vi "HFRR ADV v017 new software.vi"() -> ()   [LabVIEW 2025] (continued)
                        n2547 = Number To Fractional String(number=w3562, precision (6)=i16 2) -> (F-format string=w3561:string)  [unwired: 2 in]
                        n2548 = Concatenate Strings("Set Frequency [Hz] :" ("Content"), w3561) -> (w3564:string)
                        n2549 = local read "EVENT LOG"() -> (w3566:string)
                        n2550 = call "Event Log.vi"("Content"=w3564, "EVENT LOG"=w3566) -> ("EVENT LOG"=w3565:string)  [unwired: 8 in, 1 out]
                        n2551 = local write "EVENT LOG"(w3565) -> ()
                      }
                      frame #22 {
                        n2552 = Wait (ms)(milliseconds to wait=u32 50) -> ()  [unwired: 1 out]
                      }
                      frame #23 {
                        n2553 = local read "NORMAL LOAD"() -> (w3569:dbl)
                        n2554 = Number To Fractional String(number=w3569, precision (6)=i16 2) -> (F-format string=w3570:string)  [unwired: 2 in]
                        n2555 = Concatenate Strings("Applied Load [grams] :" ("Content"), w3570) -> (w3572:string)
                        n2556 = local read "EVENT LOG"() -> (w3574:string)
                        n2557 = call "Event Log.vi"("Content"=w3572, "EVENT LOG"=w3574) -> ("EVENT LOG"=w3573:string)  [unwired: 8 in, 1 out]
                        n2558 = local write "EVENT LOG"(w3573) -> ()
                      }
                      frame #24 {
                        n2559 = Wait (ms)(milliseconds to wait=u32 50) -> ()  [unwired: 1 out]
                      }
                      frame #25 {
                        n2560 = local read "Set Strk"() -> (w3577:dbl)
                        n2561 = Number To Fractional String(number=w3577, precision (6)=i16 2) -> (F-format string=w3578:string)  [unwired: 2 in]
                        n2562 = Concatenate Strings("Set Stroke [mm] :" ("Content"), w3578) -> (w3580:string)
                        n2563 = local read "EVENT LOG"() -> (w3582:string)
                        n2564 = call "Event Log.vi"("Content"=w3580, "EVENT LOG"=w3582) -> ("EVENT LOG"=w3581:string)  [unwired: 8 in, 1 out]
                        n2565 = local write "EVENT LOG"(w3581) -> ()
                      }
                      frame #26 {
                        n2566 = Wait (ms)(milliseconds to wait=u32 50) -> ()  [unwired: 1 out]
                      }
                      frame #27 {
                        n2567 = local read "Set Temp"() -> (w3585:dbl)
                        n2568 = Number To Fractional String(number=w3585, precision (6)=i16 2) -> (F-format string=w3586:string)  [unwired: 2 in]
                        n2569 = Concatenate Strings("Set Temperature [deg C] :" ("Content"), w3586) -> (w3588:string)
                        n2570 = local read "EVENT LOG"() -> (w3590:string)
                        n2571 = call "Event Log.vi"("Content"=w3588, "EVENT LOG"=w3590) -> ("EVENT LOG"=w3589:string)  [unwired: 8 in, 1 out]
                        n2572 = local write "EVENT LOG"(w3589) -> ()
                      }
                      frame #28 {
                        n2573 = Wait (ms)(milliseconds to wait=u32 50) -> ()  [unwired: 1 out]
                      }
                      frame #29 {
                        n2574 = local read "Set Rh"() -> (w3593:dbl)
                        n2575 = Number To Fractional String(number=w3593, precision (6)=i16 2) -> (F-format string=w3594:string)  [unwired: 2 in]
                        n2576 = Concatenate Strings("Set Humidity [%RH] :" ("Content"), w3594) -> (w3596:string)
                        n2577 = local read "EVENT LOG"() -> (w3598:string)
                        n2578 = call "Event Log.vi"("Content"=w3596, "EVENT LOG"=w3598) -> ("EVENT LOG"=w3597:string)  [unwired: 8 in, 1 out]
                        n2579 = local write "EVENT LOG"(w3597) -> ()
                      }
                      frame #30 {
                        n2580 = Wait (ms)(milliseconds to wait=u32 50) -> ()  [unwired: 1 out]
                      }
                      frame #31 {
                        n2581 = local read "test time"() -> (w3601:dbl)
                        n2582 = Number To Fractional String(number=w3601, precision (6)=i16 1) -> (F-format string=w3602:string)  [unwired: 2 in]
                        n2583 = Concatenate Strings("Test Duration [mins] :" ("Content"), w3602) -> (w3604:string)
                        n2584 = local read "EVENT LOG"() -> (w3606:string)
                        n2585 = call "Event Log.vi"("Content"=w3604, "EVENT LOG"=w3606) -> ("EVENT LOG"=w3605:string)  [unwired: 8 in, 1 out]
                        n2586 = local write "EVENT LOG"(w3605) -> ()
                      }
                      frame #32 {
                        w3607 = dbl[] [] ("History Data")
                        w3608 = cluster{"y":dbl, dbl, "y":dbl}[] [] ("History Data")
                        w3609 = FALSE ("Visible")
                        n2587 = property on="Stroke ( mm )" class="WFChart (strict)"("History Data"=w3608) -> ()  [unwired: 2 in, 2 out]
                        n2588 = property on="Humidity ( %RH )" class="WFChart (strict)"("History Data"=w3607) -> ()  [unwired: 2 in, 2 out]
                        n2589 = property on="Temperature ( Deg C )" class="WFChart (strict)"("History Data"=w3607) -> ()  [unwired: 2 in, 2 out]
                        n2590 = property on="Electrical Contact Resistance ( % )" class="WFChart (strict)"("History Data"=w3607) -> ()  [unwired: 2 in, 2 out]
                        n2591 = property on="Coefficient of Friction" class="WFChart (strict)"("History Data"=w3607) -> ()  [unwired: 2 in, 2 out]
                        n2592 = property on="Frictional Force ( N )" class="WFChart (strict)"("History Data"=w3607) -> ()  [unwired: 2 in, 2 out]
                        n2593 = property on="Coefficient of Friction" class="WFChart (strict)"("History Data"=w3607) -> ()  [unwired: 2 in, 2 out]
                        n2594 = property on="Frictional Force ( N )" class="WFChart (strict)"("History Data"=w3607) -> ()  [unwired: 2 in, 2 out]
                        n2595 = property on="Electrical Contact Resistance ( % )" class="WFChart (strict)"("History Data"=w3607) -> ()  [unwired: 2 in, 2 out]
                        n2596 = property on="Humidity ( %RH )" class="WFChart (strict)"("History Data"=w3607) -> ()  [unwired: 2 in, 2 out]
                        n2597 = property on="Stroke ( mm )" class="WFChart (strict)"("History Data"=w3608) -> ()  [unwired: 2 in, 2 out]
                        n2598 = property on="Temperature ( Deg C )" class="WFChart (strict)"("History Data"=w3607) -> ()  [unwired: 2 in, 2 out]
                        n2599 = property on="Service Password Log" class="Str"("Visible"=w3609) -> ()  [unwired: 2 in, 2 out]
                        n2600 = property on="Password 3" class="Clust (strict)"("Visible"=w3609) -> ()  [unwired: 2 in, 2 out]
                      }
                    }
                    "TEST FILE NAM,E SAVED" <- TRUE ("TEST FILE NAM,E SAVED")
                  }
                }
              }
            }
          }
        }
        n2601 = case shown="True" w2906 {
          frame False {
            n2602 = local write "tfalg"(0.0 ("tfalg")) -> ()
          }
          frame True {
            n2603 = local read "tfalg"() -> (w3051:dbl)
            n2604 = Equal?(x=w3051, y=0.0) -> (x = y?=w3052:bool)
            n2605 = case shown="True" w3052 {
              frame False {
              }
              frame True {
                n2606 = local read "Total No. of Tests"() -> (w3055:dbl)
                n2607 = local write "tfalg"(1.0 ("tfalg")) -> ()
                n2608 = local write "acq 2"(FALSE ("acq 2")) -> ()
                n2609 = Wait (ms)(milliseconds to wait=u32 200) -> ()  [unwired: 1 out]
                n2610 = Increment(x=w3055) -> (x+1=w3054:dbl)
                n2611 = local write "Total No. of Tests"(w3054) -> ()
              }
            }
          }
        }
        n2612 = local write "Test \nStatus"(w2912) -> ()
        n2613 = local write "Save"(w2912) -> ()
        n2614 = local read "Main Tab"() -> (w2869:T2)
        n2615 = case shown="True" w2893 {
          tunnel: [FALSE ("RUN") TRUE ("RUN")] -> w2892
          tunnel: [_ 1] -> w2885
          frame False {
          }
          frame True {
          }
        }
        n2616 = In Range and Coerce(upper limit=w2900, x=w2873, lower limit=w2899) -> (In Range?=w2891:bool)  [unwired: 1 out]
        n2617 = In Range and Coerce(upper limit=w2897, x=w2872, lower limit=w2898) -> (In Range?=w2889:bool)  [unwired: 1 out]
        n2618 = case shown="True" w2905 {
          frame False {
            n2619 = local read "Rt 3"() -> (w3033:bool)
            n2620 = case shown="True" w3033 {
              frame False {
              }
              frame True {
                n2621 = local write "Rt 3"(FALSE ("Rt 3")) -> ()
                n2622 = local write "Json End Flg"(TRUE ("Upld AR 2")) -> ()
              }
            }
            "Rt" <- TRUE ("Rt")
            "Rt 2" <- FALSE ("Rt")
          }
          frame True {
            n2623 = local read "Rt"() -> (w3040:bool)
            n2624 = local write "Rt 2"(TRUE ("Rt 2")) -> ()
            n2625 = case shown="True" w3040 {
              frame False {
              }
              frame True {
                w3041 = TRUE ("Upld AR 2")
                n2626 = local write "Rt"(FALSE ("Rt")) -> ()
                n2627 = local write "Upld AR"(w3041) -> ()
                n2628 = local write "Json St Flg"(w3041) -> ()
              }
            }
            "Rt 3" <- TRUE ("Rt 3")
          }
        }
        n2629 = case shown="True" w2891 {
          tunnel: [FALSE ("RUN") TRUE ("RUN")] -> w2890
          tunnel: [_ 2] -> w2884
          frame False {
          }
          frame True {
          }
        }
        n2630 = case shown="True" w2889 {
          tunnel: [FALSE ("RUN") TRUE ("RUN")] -> w2888
          tunnel: [_ 3] -> w2883
          frame False {
          }
          frame True {
          }
        }
        n2631 = case shown="\"Acquire\"" w2869 {
          tunnel: w2871 -> [_ w3102]
          frame Default {
            w3101 = 0.0 ("output")
            n2632 = local write "PID-out"(w3101) -> ()
            n2633 = local write "Frequency ( Hz )"(w3101) -> ()
          }
          frame "Acquire" {
            n2634 = stacked-sequence {
              frame #0 {
                n2635 = local read "Auto Start Test"() -> (w3104:bool)
                n2636 = case shown="True" w3104 {
                  tunnel: "RUN" -> [w3125 w3128]
                  tunnel: [w3125 w3127] -> w3105
                  frame False {
                  }
                  frame True {
                    n2637 = local read "Auto Start Temp"() -> (w3126:bool)
                    n2638 = Or(x=w3128, y=w3126) -> (x .or. y?=w3127:bool)
                  }
                }
                n2639 = local read "clk"() -> (w3124:dbl)
                n2640 = local read "Save"() -> (w3120:bool)
                n2641 = Equal?(x=w3124, y=0.0) -> (x = y?=w3121:bool)
                n2642 = And(x=w3121, y=w3120) -> (x .and. y?=w3122:bool)
                n2643 = Not(x="Engage") -> (.not. x?=w3111:bool)
                n2644 = case shown="False" w3105 {
                  tunnel: [0.0 w3151] -> w3107
                  frame False {
                    (unwired) TRUE ("Visible")
                    n2645 = local read "Auto Start Test"() -> (w3132:bool)
                    n2646 = local write "Start Time"(TRUE ("Start Time")) -> ()
                    n2647 = property on="Stroke 2" class="DigNum (strict)"("Visible"=FALSE) -> ()  [unwired: 2 in, 2 out]
                    n2648 = case shown="False" w3132 {
                      frame False {
                        n2649 = property on="Heater Button" class="Bool (strict)"("DisabledEnum"=T19."Enabled" ("Disabled")) -> ()  [unwired: 2 in, 2 out]
                        n2650 = property on="Humidity" class="Bool (strict)"("DisabledEnum"=T19."Enabled" ("Disabled")) -> ()  [unwired: 2 in, 2 out]
                      }
                      frame True {
                      }
                    }
                    n2651 = case shown="False" "TestCompFlg" {
                      frame False {
                        n2652 = local read "StartFlg"() -> (w3140:bool)
                        n2653 = case shown="True" w3140 {
                          frame False {
                          }
                          frame True {
                            n2654 = stacked-sequence {
                              frame #0 {
                                n2655 = local read "EVENT LOG"() -> (w3144:string)
                                n2656 = call "Event Log.vi"("Content"="Test was interrupted", "EVENT LOG"=w3144) -> ("EVENT LOG"=w3145:string)  [unwired: 8 in, 1 out]
                                n2657 = local write "EVENT LOG"(w3145) -> ()
                                n2658 = property on="RUN" class="Bool (strict)"("Visible"=TRUE) -> ()  [unwired: 2 in, 2 out]
                                n2659 = property on="Auto Start Test" class="Bool (strict)"("Visible"=TRUE) -> ()  [unwired: 2 in, 2 out]
                              }
                              frame #1 {
                                w3147 = FALSE ("StartFlg")
                                n2660 = property on="Heater Button" class="Bool (strict)"("Val(Sgnl)"=FALSE ("Value (Signaling)")) -> ()  [unwired: 2 in, 2 out]
                                n2661 = local write "Heater Button"(w3147) -> ()
                                n2662 = local write "StartFlg"(w3147) -> ()
                                n2663 = local write "Humidity"(w3147) -> ()
                              }
                              frame #2 {
                                n2664 = local write "Command"("VC;0" ("Command")) -> ()
                              }
                              frame #3 {
                                n2665 = Wait (ms)(milliseconds to wait=u32 1500) -> ()  [unwired: 1 out]
                              }
                              frame #4 {
                                n2666 = local write "Command"("HE;0" ("Command")) -> ()
                              }
                            }
                          }
                        }
                      }
                      frame True {
                      }
                    }
                    n2667 = local write "String 14"("Test will autostart once parameters reach the set value." ("String 14")) -> ()
                  }
                  frame True {
                    (unwired) FALSE ("Visible")
                    n2668 = property on="Stroke 2" class="DigNum (strict)"("Visible"=TRUE) -> ()  [unwired: 2 in, 2 out]
                    n2669 = property on="STOP 2" class="Bool (strict)"("Disabled"=u8 2) -> ()  [unwired: 2 in, 2 out]
                    n2670 = local write "String 14"(" Running....." ("String 14")) -> ()
                    n2671 = property on="Heater Button" class="Bool (strict)"("DisabledEnum"=T19."Disabled and Grayed Out" ("Disabled")) -> ()  [unwired: 2 in, 2 out]
                    n2672 = property on="Humidity" class="Bool (strict)"("DisabledEnum"=T19."Disabled and Grayed Out" ("Disabled")) -> ()  [unwired: 2 in, 2 out]
                    n2673 = case shown="True" "Start Time" {
                      selector: "Start Time" -> [_ w3170]
                      frame False {
                      }
                      frame True {
                        n2674 = Not(x=w3170) -> (.not. x?=w3169:bool)
                        n2675 = local write "Start Time"(w3169) -> ()
                        n2676 = local read "EVENT LOG"() -> (w3171:string)
                        n2677 = call "Event Log.vi"("Content"="Test in progress", "EVENT LOG"=w3171) -> ("EVENT LOG"=w3173:string)  [unwired: 8 in, 1 out]
                        n2678 = local write "EVENT LOG"(w3173) -> ()
                      }
                    }
                    n2679 = disable-structure shown="Enabled" {
                      disable-tunnel: [w3162 w3168] -> w3151
                      frame Disabled {
                        n2680 = local read "Set Hz"() -> (w3165:dbl)
                        n2681 = call <vilib>:"Uniform White Noise Waveform.vi"() -> ("signal out"=w3164:waveform(dbl))  [unwired: 10 in, 1 out]
                        n2682 = Random Number (0-1)() -> (number: 0 to 1=w3161:dbl)
                        n2683 = Add(x=w3165, y=w3164) -> (x+y=w3163:waveform(dbl))
                        n2684 = Multiply(x=ext 0.01 ("y"), y=w3161) -> (x*y=w3159:ext)
                        n2685 = Multiply(x=w3163, y=w3159) -> (x*y=w3162:waveform(ext))
                      }
                      frame Enabled {
                        n2686 = call-poly <vilib>:"Random Number (Range).vi"("lower bound (0)"=49.89, "upper bound (100)"=50.8) -> ("number"=w3168:dbl)  [unwired: 9 in]
                      }
                    }
                    "StartFlg" <- TRUE ("StartFlg")
                  }
                }
                n2687 = case shown="True" w3122 {
                  frame False {
                  }
                  frame True {
                    n2688 = local write "clk"(10.0 ("clk")) -> ()
                    n2689 = Get Date/Time In Seconds() -> (seconds since 1Jan1904=w3176:timestamp)
                    n2690 = To Double Precision Float(number=w3176) -> (double precision float=w3174:dbl)
                    n2691 = local write "acq timer"(w3174) -> ()
                    n2692 = local write "act save time"(w3174) -> ()
                  }
                }
                n2693 = call "Elapsed Time"("Time Target (s)"="Countdown", "Reset"=w3111) -> ("Elapsed Time (s)"=w3116:dbl, "Time has Elapsed"=w3114:bool)  [unwired: 10 in, 6 out]
                "Countdown 2" <- w3116
                n2694 = Subtract(x=w3116, y=2.0) -> (x-y=w3119:dbl)
                n2695 = Less?(x=w3119, y="Countdown") -> (x < y?=w3117:bool)
                n2696 = And(x=w3117, y=w3114) -> (x .and. y?=w3113:bool)
                n2697 = case shown="True" w3113 {
                  frame False {
                  }
                  frame True {
                    (unwired) dbl[] [] ("History Data")
                    n2698 = local write "Engage"(FALSE ("Engage")) -> ()
                    n2699 = local write "RUN"(TRUE ("RUN")) -> ()
                    n2700 = local read "Humidity ( %RH )"() -> (→"Rh Before":dbl)
                  }
                }
                n2701 = local read "Test \nStatus"() -> (w3109:bool)
                n2702 = Select(t=w3107, s=w3109, f=0.0) -> (s? t:f=w3108:dbl)
                n2703 = local write "Frequency ( Hz )"(w3108) -> ()
              }
              frame #1 {
                w3199 = 1000000.0 ("x")
                # "HC;1/0\nST;VALUE"
                # "Elapsed time\ncof\nstroke\nAir temp\nTemp\nHumidity"
                # "acq timer\n\nact save time"
                # "convert to microseconds"
                n2704 = local read "COUNT"() -> (w3182:i32)
                n2705 = local read "Rate"() -> (w3195:dbl)
                n2706 = Divide(x=w3199, y=w3195) -> (x/y=w3200:dbl)
                n2707 = Greater Or Equal?(x=w3182, y=250) -> (x >= y?=w3181:bool)
                n2708 = Get Date/Time In Seconds() -> (seconds since 1Jan1904=w3202:timestamp)
                n2709 = case shown="True" w3181 {
                  frame False {
                    n2710 = local read "COUNT"() -> (w3203:i32)
                    n2711 = Increment(x=w3203) -> (x+1=w3204:i32)
                    n2712 = local write "COUNT"(w3204) -> ()
                  }
                  frame True {
                    n2713 = local write "COUNT"(0 ("COUNT")) -> ()
                  }
                }
                n2714 = local read "Samplingtime 2"() -> (w3180:dbl)
                n2715 = local read "act save time"() -> (w3197:dbl)
                n2716 = Divide(x=w3200, y=w3199) -> (x/y=w3198:dbl)
                n2717 = To Double Precision Float(number=w3202) -> (double precision float=w3191:dbl)
                n2718 = Add(x=w3197, y=w3180) -> (x+y=w3196:dbl)
                n2719 = local read "acq timer"() -> (w3201:dbl)
                n2720 = local read "COUNT"() -> (w3184:i32)
                n2721 = Greater Or Equal?(x=w3191, y=w3196) -> (x >= y?=w3179:bool)
                n2722 = Multiply(x=w3198, y=w3184) -> (x*y=w3190:dbl)
                n2723 = Subtract(x=w3191, y=w3201) -> (x-y=w3193:dbl)
                n2724 = local read "Save"() -> (w3194:bool)
                n2725 = Add(x=w3193, y=w3190) -> (x+y=w3177:dbl)
                "Elapsed time 3" <- w3177
                n2726 = And(x=w3179, y=w3194) -> (x .and. y?=w3192:bool)
                n2727 = Divide(x=w3177, y=60.0) -> (x/y=w3188:dbl)
                n2728 = local read "Test \nStatus"() -> (w3178:bool)
                n2729 = local read "clk"() -> (w3185:dbl)
                n2730 = Equal?(x=w3185, y=10.0) -> (x = y?=w3187:bool)
                n2731 = case shown="True" w3192 {
                  tunnel: w3191 -> [_ w3315]
                  tunnel: [FALSE ("Boolean 2") TRUE ("Boolean 2")] -> _
                  frame False {
                  }
                  frame True {
                    w3269 = ";" ("Substring")
                    # "Pid out/\nFreq response value"
                    n2732 = local write "act save time"(w3315) -> ()
                    n2733 = local read "FILE"() -> (w3263:string)
                    n2734 = call "file check.vi"("file name in"=w3263) -> ("error out"=w3266:errorcluster, "file name out"=w3261:string)  [unwired: 9 in]
                    n2735 = local read "LVDT STROKE"() -> (w3258:dbl)
                    n2736 = local read "Add up Stroke"() -> (w3256:dbl)
                    n2737 = call "FILE PATH CREATION.vi"("error in"=w3266, "FILE NAME :"=w3261) -> ("FILE OUT"=w3264:path)  [unwired: 8 in, 1 out]
                    n2738 = Concatenate Strings(w3261, ".dgf" ("Substring")) -> (w3265:string)
                    n2739 = Subtract(x=w3258, y=w3256) -> (x-y=w3257:dbl)
                    n2740 = Absolute Value(x=w3257) -> (abs(x)=w3255:dbl)
                    n2741 = local read "FF 2"() -> (→"Frictional Force ( N )" →"Frictional Force ( N )":dbl)
                    n2742 = Build Path(base path=w3264, name or relative path=w3265) -> (appended path=w3260:path)
                    n2743 = local read "COF 2"() -> (w3274:dbl)
                    "cof" <- w3274
                    "Coefficient of Friction" <- w3274
                    "COF 4" <- w3274
                    "Coefficient of Friction" <- w3274
                    n2744 = local read "TEMP"() -> (w3277:dbl)
                    "Temp" <- w3277
                    "Temperature ( Deg C )" <- w3277
                    n2745 = local read "Humidity ( %RH )"() -> (w3276:dbl)
                    "Humidity ( %RH )" <- w3276
                    "Humidity ( %RH )" <- w3276
                    n2746 = local read "Frequency ( Hz )"() -> (w3283:dbl)
                    n2747 = call <vilib>:"Mean PtByPt.vi"("x"=w3255, "sample length"="STROKE FILTER") -> ("mean"=w3254:dbl)  [unwired: 2 in, 1 out]
                    n2748 = local read "Elapsed time"() -> (w3308:dbl)
                    n2749 = local read "AIR TEMP"() -> (w3281:dbl)
                    n2750 = local read "PID-out"() -> (w3286:dbl)
                    n2751 = local write "Temperature ( Deg C )"(w3277) -> ()
                    n2752 = Number To Fractional String(number=w3254, width (-)=i16 9 ("precision (6)"), precision (6)=i16 6) -> (F-format string=w3301:string)  [unwired: 1 in]
                    n2753 = Number To Fractional String(number=w3281, width (-)=i16 9 ("precision (6)"), precision (6)=i16 3) -> (F-format string=w3300:string)  [unwired: 1 in]
                    n2754 = Number To Fractional String(number=w3277, width (-)=i16 9 ("precision (6)"), precision (6)=i16 3) -> (F-format string=w3297:string)  [unwired: 1 in]
                    n2755 = Number To Fractional String(number=w3276, width (-)=i16 9 ("precision (6)"), precision (6)=i16 3) -> (F-format string=w3294:string)  [unwired: 1 in]
                    n2756 = Number To Fractional String(number=0.0, width (-)=i16 9 ("precision (6)"), precision (6)=i16 3) -> (F-format string=w3291:string)  [unwired: 1 in]
                    n2757 = Number To Fractional String(number=w3286, width (-)=i16 9 ("precision (6)"), precision (6)=i16 3) -> (F-format string=w3287:string)  [unwired: 1 in]
                    n2758 = Number To Fractional String(number=w3283, width (-)=i16 9 ("precision (6)"), precision (6)=i16 3) -> (F-format string=w3282:string)  [unwired: 1 in]
                    n2759 = Number To Fractional String(number=w3274, width (-)=i16 9 ("precision (6)"), precision (6)=i16 6) -> (F-format string=w3309:string)  [unwired: 1 in]
                    n2760 = Number To Fractional String(number=w3308, width (-)=i16 14 ("precision (6)"), precision (6)=i16 3) -> (F-format string=w3310:string)  [unwired: 1 in]
                    n2761 = Bundle("y"=1.02, "mean"=w3254, "y"=0.98) -> (w3275:cluster{"y":dbl, "mean":dbl, "y":dbl})  [unwired: 1 in]
                    n2762 = Number To Fractional String(number="Ambient Humidity :", width (-)=i16 9 ("precision (6)"), precision (6)=i16 6) -> (F-format string=w3267:string)  [unwired: 1 in]
                    n2763 = local read "RUN"() -> (w3273:bool)
                    n2764 = case shown="True" w3273 {
                      tunnel: w3275 -> [_ w3320]
                      tunnel: w3254 -> [_ w3319]
                      tunnel: w3254 -> [_ w3317]
                      tunnel: w3254 -> [_ w3318]
                      frame False {
                      }
                      frame True {
                        "Stroke ( mm )" <- w3320
                        "Stroke ( mm )" <- w3320
                        "Stroke 4" <- w3319
                        "Stroke 3" <- w3317
                        "Stroke 2" <- w3318
                        "measured_stroke" <- w3317
                      }
                    }
                    n2765 = Concatenate Strings(w3310, w3269, w3309, w3269, w3301, w3269, w3300, w3269, w3297, w3269, w3294, w3269, w3291, w3269, w3287, w3269, w3282, w3269, w3267, "\r") -> (w3307:string)
                    n2766 = call <vilib>:"Write Characters To File.vi"("append to file? (new file:F)"=TRUE, "character string"=w3307, "file path (dialog if empty)"=w3260) -> ()  [unwired: 2 in, 1 out]
                    "refresh flag" <- TRUE ("refresh flag")
                  }
                }
                n2767 = case shown="True" w3178 {
                  tunnel: w3188 -> [_ w3214]
                  tunnel: w3193 -> [_ w3224]
                  tunnel: [0.0 w3220] -> _
                  tunnel: w3187 -> [_ w3219]
                  tunnel: [0.0 w3218] -> _
                  tunnel: w3177 -> [_ w3218]
                  tunnel: w3191 -> [w3207 _]
                  frame False {
                    n2768 = local write "acq timer"(w3207) -> ()
                    n2769 = local write "Test Duration Status"(0.0 ("Test Duration Status")) -> ()
                  }
                  frame True {
                    n2770 = local read "Set Hz"() -> (w3221:dbl)
                    n2771 = local write "Elapsed time"(w3214) -> ()
                    n2772 = local read "test time"() -> (w3213:dbl)
                    n2773 = Multiply(x=w3224, y=w3221) -> (x*y=w3223:dbl)
                    n2774 = case shown="False" w3219 {
                      tunnel: w3223 -> [w3225 _]
                      tunnel: [w3225 1.0] -> w3220
                      frame False {
                        n2775 = local write "Cycles elapsed"(w3225) -> ()
                      }
                      frame True {
                      }
                    }
                    n2776 = Greater?(x=w3214, y=w3213) -> (0:w3222:bool)
                    n2777 = Subtract(x=w3213, y=w3214) -> (x-y=w3212:dbl)
                    "time" <- w3212
                    n2778 = Multiply(x=w3212, y=60.0) -> (x*y=w3211:dbl)
                    n2779 = local write "Time Remaining"(w3211) -> ()
                    n2780 = local write "Remaining Time"(w3211) -> ()
                    n2781 = case shown="True" w3222 {
                      frame False {
                      }
                      frame True {
                        n2782 = stacked-sequence {
                          frame #0 {
                            w3230 = T19."Enabled" ("Disabled")
                            w3229 = FALSE ("TEST FILE NAM,E SAVED")
                            w3231 = "" ("FILE")
                            w3232 = TRUE ("Visible")
                            n2783 = local write "Humidity"(FALSE ("Humidity")) -> ()
                            n2784 = local write "RUN"(FALSE ("OK Button 2")) -> ()
                            n2785 = local write "Heater Button"(FALSE ("Heater Button")) -> ()
                            n2786 = local write "Auto Start Test"(FALSE ("Auto Start Test")) -> ()
                            n2787 = local write "TestCompFlg"(TRUE ("StpFlg")) -> ()
                            n2788 = local read "Humidity ( %RH )"() -> (→"Rh After":dbl)
                            n2789 = property on="STOP 2" class="Bool (strict)"("Disabled"=u8 0) -> ()  [unwired: 2 in, 2 out]
                            n2790 = local read "EVENT LOG"() -> (w3237:string)
                            n2791 = call "Event Log.vi"("Content"="Test Completed", "EVENT LOG"=w3237) -> ("EVENT LOG"=w3236:string)  [unwired: 8 in, 1 out]
                            n2792 = property on="RUN" class="Bool (strict)"("Visible"=w3232) -> ()  [unwired: 2 in, 2 out]
                            n2793 = property on="Auto Start Test" class="Bool (strict)"("Visible"=w3232) -> ()  [unwired: 2 in, 2 out]
                            n2794 = local write "Batch Ref Num :"(w3231) -> ()
                            n2795 = local write "FILE"(w3231) -> ()
                            n2796 = local write "EVENT LOG"(w3236) -> ()
                            n2797 = local write "TEST FILE NAM,E SAVED"(w3229) -> ()
                            n2798 = local write "Fuel Discription :"(w3231) -> ()
                            n2799 = local write "START TEMP"(w3229) -> ()
                            n2800 = local write "Remarks :"(w3231) -> ()
                            n2801 = local write "Main Dashboard Buttons"(T1."Imaging" ("Main Dashboard Buttons")) -> ()
                            n2802 = local write "Main Tab"(T2."Adv Scar" ("Main Tab")) -> ()
                            n2803 = property on="FRICVALZ 2" class="Bool (strict)"("DisabledEnum"=w3230) -> ()  [unwired: 2 in, 2 out]
                            n2804 = property on="FRICVALZ 3" class="Bool (strict)"("DisabledEnum"=w3230) -> ()  [unwired: 2 in, 2 out]
                            n2805 = property on="FRICVALZ 4" class="Bool (strict)"("DisabledEnum"=w3230) -> ()  [unwired: 2 in, 2 out]
                          }
                          frame #1 {
                            n2806 = Wait (ms)(milliseconds to wait=u32 1500) -> ()  [unwired: 1 out]
                          }
                          frame #2 {
                            n2807 = local write "Command"("VC;0") -> ()
                          }
                          frame #3 {
                            n2808 = Wait (ms)(milliseconds to wait=u32 1500) -> ()  [unwired: 1 out]
                          }
                          frame #4 {
                            n2809 = local write "Command"("VC;0") -> ()
                          }
                          frame #5 {
                            n2810 = Wait (ms)(milliseconds to wait=u32 1500) -> ()  [unwired: 1 out]
                          }
                          frame #6 {
                            n2811 = local write "Command"("ST;0") -> ()
                          }
                          frame #7 {
                            n2812 = local write "measured_stroke"(0.0 ("measured_stroke")) -> ()
                            n2813 = Wait (ms)(milliseconds to wait=u32 1500) -> ()  [unwired: 1 out]
                          }
                          frame #8 {
                            n2814 = local write "Command"("HE;0") -> ()
                          }
                        }
                      }
                    }
                    n2815 = Divide(x=w3214, y=w3213) -> (x/y=w3217:dbl)
                    n2816 = Multiply(x=w3217, y=100.0) -> (x*y=w3215:dbl)
                    n2817 = local write "Test Duration Status"(w3215) -> ()
                  }
                }
              }
              frame #2 {
                n2818 = case shown="True" "Heater Button" {
                  tunnel: [0.0 ("output") w3343] -> w3321
                  frame False {
                    w3324 = TRUE ("tmpchk")
                    n2819 = local read "TEMP"() -> (w3325:dbl)
                    n2820 = local write "Temp ini"(w3325) -> ()
                    n2821 = local write "Reset 4"(w3324) -> ()
                    n2822 = local write "tmpchk"(w3324) -> ()
                    n2823 = local write "reinit"(TRUE ("reinit")) -> ()
                    n2824 = local write "manual temp log"(TRUE ("manual temp log")) -> ()
                  }
                  frame True {
                    # "Logic to turn off\nthe heater when \ntemp is not rising.\nTime - 60 sec\nDelta t- 5°c"
                    n2825 = local read "Temp ini"() -> (w3332:dbl)
                    n2826 = local read "Auto Start Test"() -> (w3328:bool)
                    n2827 = Less?(x=w3332, y=53.0) -> (x < y?=w3330:bool)
                    n2828 = case shown="False" w3328 {
                      frame False {
                        n2829 = local read "Set Temp"() -> (w3352:dbl)
                        n2830 = local read "TEMP"() -> (w3351:dbl)
                        n2831 = Subtract(x=w3352, y=w3351) -> (x-y=w3350:dbl)
                        n2832 = Absolute Value(x=w3350) -> (abs(x)=w3349:dbl)
                        n2833 = Less?(x=w3349, y=0.5) -> (x < y?=w3347:bool)
                        n2834 = case shown="True" w3347 {
                          tunnel: "manual temp log" -> [_ w3353]
                          frame False {
                          }
                          frame True {
                            n2835 = case shown="True" w3353 {
                              selector: w3353 -> [_ w3354]
                              frame False {
                              }
                              frame True {
                                # "#Event log"
                                n2836 = Not(x=w3354) -> (.not. x?=w3355:bool)
                                n2837 = local write "manual temp log"(w3355) -> ()
                                n2838 = local read "EVENT LOG"() -> (w3358:string)
                                n2839 = call "Event Log.vi"("Content"="Target Temperature reached", "EVENT LOG"=w3358) -> ("EVENT LOG"=w3357:string)  [unwired: 8 in, 1 out]
                                n2840 = local write "EVENT LOG"(w3357) -> ()
                              }
                            }
                          }
                        }
                      }
                      frame True {
                        n2841 = local write "manual temp log"(TRUE ("manual temp log")) -> ()
                      }
                    }
                    n2842 = And(x="tmpchk", y=w3330) -> (x .and. y?=w3333:bool)
                    n2843 = case shown="True" w3333 {
                      frame False {
                      }
                      frame True {
                        n2844 = call "Elapsed Time8"("Time Target (s)"=300.0, "Reset"="Reset 4") -> ("Time has Elapsed"=w3360:bool)  [unwired: 10 in, 7 out]
                        n2845 = flat-sequence {
                          tunnel: w3360 -> [_]
                          frame #0 {
                            n2846 = local write "Reset 4"(FALSE ("Reset 4")) -> ()
                          }
                        }
                        n2847 = case shown="True" w3360 {
                          frame False {
                          }
                          frame True {
                            n2848 = local read "Temp ini"() -> (w3367:dbl)
                            n2849 = Add(x=w3367, y=5.0) -> (x+y=w3365:dbl)
                            n2850 = local read "TEMP"() -> (w3368:dbl)
                            n2851 = Greater?(x=w3368, y=w3365) -> (0:w3366:bool)
                            n2852 = case shown="False" w3366 {
                              frame False {
                                n2853 = local write "Heater Button"(FALSE ("Heater Button")) -> ()
                              }
                              frame True {
                                n2854 = local write "tmpchk"(FALSE ("tmpchk")) -> ()
                              }
                            }
                          }
                        }
                      }
                    }
                    n2855 = local read "Set Temp"() -> (w3341:dbl)
                    n2856 = local read "TEMP"() -> (w3335:dbl)
                    n2857 = call-poly <vilib>:"PID.vi"("reinitialize? (F)"="reinit", "dt (s)"=-1.0, "process variable"=w3335, "setpoint"=w3341) -> ("output"=w3338:dbl)  [unwired: 6 in, 1 out]
                    n2858 = Subtract(x=w3341, y=w3335) -> (x-y=w3342:dbl)
                    n2859 = Add(x=w3341, y=0.5) -> (x+y=w3339:dbl)
                    n2860 = Greater Or Equal?(x=w3335, y=w3339) -> ()  [unwired: 1 out]
                    n2861 = Select(t=0.0, s=FALSE, f=w3338) -> (s? t:f=w3337:dbl)
                    "PID output" <- w3337
                    n2862 = flat-sequence {
                      tunnel: w3337 -> [w3371]
                      tunnel: [w3371] -> w3343
                      frame #0 {
                        n2863 = local write "reinit"(FALSE ("reinit")) -> ()
                      }
                    }
                    n2864 = Bundle(w3342, "output"=w3337, "TEMP"=w3335) -> ()  [unwired: 1 in, 1 out]
                  }
                }
                "PID-out" <- w3321
              }
              frame #3 {
                n2865 = local read "TEMP"() -> (w3373:dbl)
                n2866 = Greater Or Equal?(x=w3373, y="Set Temp 2") -> (x >= y?=w3378:bool)
                n2867 = case shown="True" w3378 {
                  tunnel: [FALSE TRUE] -> w3376
                  frame False {
                  }
                  frame True {
                  }
                }
                "Status 13" <- w3376
                n2868 = And(x=w3376, y="trip1 8") -> (x .and. y?=w3375:bool)
                n2869 = case shown="True" w3375 {
                  frame False {
                    n2870 = local write "Heater Trip Temp"(TRUE ("Heater Trip Temp")) -> ()
                  }
                  frame True {
                    w3381 = FALSE ("OK Button 2")
                    n2871 = case shown="True" "Heater Trip Temp" {
                      selector: "Heater Trip Temp" -> [_ w3383]
                      frame False {
                      }
                      frame True {
                        n2872 = Not(x=w3383) -> (.not. x?=w3382:bool)
                        n2873 = local read "EVENT LOG"() -> (w3386:string)
                        n2874 = local write "Heater Trip Temp"(w3382) -> ()
                        n2875 = call "Event Log.vi"("Content"="Heater Trip", "EVENT LOG"=w3386) -> ("EVENT LOG"=w3385:string)  [unwired: 8 in, 1 out]
                        n2876 = local write "EVENT LOG"(w3385) -> ()
                      }
                    }
                    n2877 = local write "RUN"(w3381) -> ()
                    n2878 = property on="Auto Start Test" class="Bool (strict)"("Value"=w3381) -> ()  [unwired: 2 in, 2 out]
                    n2879 = local write "Heater Button"(w3381) -> ()
                  }
                }
              }
            }
            n2880 = case shown="False" w3102 {
              frame False {
                n2881 = disable-structure shown="Disabled" {
                  frame Disabled {
                    n2882 = stacked-sequence {
                      frame #0 {
                        n2883 = local write "RUN"(FALSE ("OK Button 2")) -> ()
                      }
                      frame #1 {
                      }
                    }
                  }
                  frame Enabled {
                  }
                }
              }
              frame True {
              }
            }
          }
        }
        n2884 = local read "airtempflg"() -> (w2894:bool)
        n2885 = Or(x=w2894, y=w2892) -> (x .or. y?=w2895:bool)
        n2886 = Insert Into Array(array=string[] ["Air Temperature has reached set value,", "Humidity has reached set value,", "Sample Temperaturehas reached set value,", ""], index=0, new element="") -> (w2880:string[])
        n2887 = Build Array(w2885, w2884, w2883) -> (w2881:i32[])
        n2888 = disable-structure shown="Disabled" {
          disable-tunnel: w2895 -> [w2972 _]
          disable-tunnel: w2890 -> [w2971 _]
          disable-tunnel: w2888 -> [w2970 _]
          frame Disabled {
            n2889 = Compound Arithmetic op=AND(w2972, w2971, w2970) -> ()  [unwired: 1 out]
            n2890 = case shown="True" {
              selector: _ -> [_ _]
              frame False {
              }
              frame True {
                w2973 = FALSE ("autostrtflg")
                n2891 = local write "RUN"(TRUE ("RUN")) -> ()
                n2892 = local write "autostrtflg"(w2973) -> ()
                n2893 = local write "autostart"(w2973) -> ()
                n2894 = local write "String 14"(" Running....." ("String 14")) -> ()
              }
            }
          }
          frame Enabled {
          }
        }
        n2895 = for {
          tunnel: w2881 -> [w3023] mode=indexing
          tunnel: w2880 -> [w3022]
          shift-right: [w3019] -> w2879
          shift-left: "" -> [w3021]
          n2896 = Index Array(array=w3022, index=w3023) -> (element=w3020:string)
          n2897 = Concatenate Strings(w3020, w3021) -> (w3019:string)
        }
        n2898 = local write "autostart 2"(w2879) -> ()
        n2899 = local read "Reset Graph"() -> (w2868:bool)
        n2900 = case shown="True" w2868 {
          selector: w2868 -> [_ w2922]
          frame False {
          }
          frame True {
            w2936 = 0.0 ("X Scale.Range:Maximum")
            n2901 = Not(x=w2922) -> (.not. x?=w2921:bool)
            n2902 = local write "Reset Graph"(w2921) -> ()
            n2903 = property on="Electrical Contact Resistance ( % )" class="WFChart (strict)"("XScale.Maximum"=600.0 ("X Scale.Range:Maximum"), "XScale.Minimum"=0.0 ("X Scale.Range:Minimum"), "YScale.Maximum"=100.0 ("Y Scale.Range:Maximum"), "YScale.Minimum"=0.0 ("Y Scale.Range:Minimum")) -> ()  [unwired: 2 in, 2 out]
            n2904 = property on="Frictional Force ( N )" class="WFChart (strict)"("XScale.Maximum"=600.0 ("X Scale.Range:Maximum"), "XScale.Minimum"=0.0 ("X Scale.Range:Minimum"), "YScale.Maximum"=100.0 ("Y Scale.Range:Maximum"), "YScale.Minimum"=0.0 ("Y Scale.Range:Minimum")) -> ()  [unwired: 2 in, 2 out]
            n2905 = property on="Temperature ( Deg C )" class="WFChart (strict)"("XScale.Maximum"=600.0 ("X Scale.Range:Maximum"), "XScale.Minimum"=0.0 ("X Scale.Range:Minimum"), "YScale.Maximum"=100.0 ("Y Scale.Range:Maximum"), "YScale.Minimum"=0.0 ("Y Scale.Range:Minimum")) -> ()  [unwired: 2 in, 2 out]
            n2906 = property on="Humidity ( %RH )" class="WFChart (strict)"("XScale.Maximum"=600.0 ("X Scale.Range:Maximum"), "XScale.Minimum"=0.0 ("X Scale.Range:Minimum"), "YScale.Maximum"=100.0 ("Y Scale.Range:Maximum"), "YScale.Minimum"=0.0 ("Y Scale.Range:Minimum")) -> ()  [unwired: 2 in, 2 out]
            n2907 = property on="Stroke ( mm )" class="WFChart (strict)"("XScale.Maximum"=600.0 ("X Scale.Range:Maximum"), "XScale.Minimum"=0.0 ("X Scale.Range:Minimum"), "YScale.Maximum"=100.0 ("Y Scale.Range:Maximum"), "YScale.Minimum"=0.0 ("Y Scale.Range:Minimum")) -> ()  [unwired: 2 in, 2 out]
            n2908 = property on="Coefficient of Friction" class="WFChart (strict)"("XScale.Maximum"=600.0 ("X Scale.Range:Maximum"), "XScale.Minimum"=0.0 ("X Scale.Range:Minimum"), "YScale.Maximum"=100.0 ("Y Scale.Range:Maximum"), "YScale.Minimum"=0.0 ("Y Scale.Range:Minimum")) -> ()  [unwired: 2 in, 2 out]
            n2909 = property on="Electrical Contact Resistance ( % )" class="WFChart (strict)"("XScale.Minimum"=0.0 ("X Scale.Range:Minimum"), "XScale.Maximum"=600.0 ("X Scale.Range:Maximum"), "YScale.Minimum"=0.0 ("Y Scale.Range:Minimum"), "YScale.Maximum"=100.0 ("Y Scale.Range:Maximum")) -> ()  [unwired: 2 in, 2 out]
            n2910 = property on="Temperature ( Deg C )" class="WFChart (strict)"("XScale.Minimum"=0.0 ("X Scale.Range:Minimum"), "XScale.Maximum"=600.0 ("X Scale.Range:Maximum"), "YScale.Minimum"=0.0 ("Y Scale.Range:Minimum"), "YScale.Maximum"=100.0 ("Y Scale.Range:Maximum")) -> ()  [unwired: 2 in, 2 out]
            n2911 = property on="Coefficient of Friction" class="WFChart (strict)"("XScale.Minimum"=0.0 ("X Scale.Range:Minimum"), "XScale.Maximum"=600.0 ("X Scale.Range:Maximum"), "YScale.Maximum"=1.0 ("X Scale.Range:Minimum"), "YScale.Minimum"=0.0 ("X Scale.Range:Minimum")) -> ()  [unwired: 2 in, 2 out]
            n2912 = property on="Frictional Force ( N )" class="WFChart (strict)"("XScale.Maximum"=600.0 ("X Scale.Range:Maximum"), "XScale.Minimum"=w2936, "YScale.Maximum"=10.0 ("Y Scale.Range:Maximum"), "YScale.Minimum"=w2936) -> ()  [unwired: 2 in, 2 out]
            n2913 = property on="Stroke ( mm )" class="WFChart (strict)"("XScale.Maximum"=600.0 ("X Scale.Range:Maximum"), "XScale.Minimum"=0.0 ("X Scale.Range:Minimum"), "YScale.Maximum"=100.0 ("Y Scale.Range:Maximum"), "YScale.Minimum"=0.0 ("Y Scale.Range:Minimum")) -> ()  [unwired: 2 in, 2 out]
            n2914 = property on="Humidity ( %RH )" class="WFChart (strict)"("XScale.Maximum"=600.0 ("X Scale.Range:Maximum"), "XScale.Minimum"=0.0 ("X Scale.Range:Minimum"), "YScale.Maximum"=100.0 ("Y Scale.Range:Maximum"), "YScale.Minimum"=0.0 ("Y Scale.Range:Minimum")) -> ()  [unwired: 2 in, 2 out]
          }
        }
      }
      frame "Compare Files" {
        # "Elapsed time\ncof\nstroke\nAir temp\nTemp\nHumidity"
        n2915 = case shown="True" "RSTV1 2" {
          frame False {
          }
          frame True {
            n2916 = property on="Humidity ( %RH )" class="XYGraph (strict)"("Y Scale.Display Format:Precision"=u8 0 ("Y Scale.Format & Precision:Precision")) -> ()  [unwired: 2 in, 2 out]
            n2917 = property on="Humidity ( %RH )" class="XYGraph (strict)"("X Scale.Range:Minimum"=0.0, "X Scale.Range:Maximum"=75.0, "Y Scale.Range:Minimum"=48.0, "Y Scale.Range:Maximum"=58.0) -> ()  [unwired: 2 in, 2 out]
          }
        }
        n2918 = case shown="True" "RST CP 2" {
          frame False {
          }
          frame True {
            n2919 = property on="XY Graph 13" class="XYGraph (strict)"("Y Scale.Display Format:Precision"=u8 0 ("Y Scale.Format & Precision:Precision")) -> ()  [unwired: 2 in, 2 out]
            n2920 = property on="XY Graph 13" class="XYGraph (strict)"("X Scale.Range:Minimum"=0.0, "X Scale.Range:Maximum"=75.0, "Y Scale.Range:Minimum"=0.0, "Y Scale.Range:Maximum"=100.0) -> ()  [unwired: 2 in, 2 out]
          }
        }
        n2921 = case shown="True" "RST CP" {
          frame False {
          }
          frame True {
            n2922 = property on="Sample Temperature ( °C )" class="XYGraph (strict)"("Y Scale.Display Format:Precision"=u8 2 ("Y Scale.Format & Precision:Precision")) -> ()  [unwired: 2 in, 2 out]
            n2923 = property on="Sample Temperature ( °C )" class="XYGraph (strict)"("X Scale.Range:Minimum"=0.0, "X Scale.Range:Maximum"=75.0, "Y Scale.Range:Minimum"=58.0, "Y Scale.Range:Maximum"=62.0) -> ()  [unwired: 2 in, 2 out]
          }
        }
        n2924 = case shown="True" "RSTV1 3" {
          frame False {
          }
          frame True {
            n2925 = property on="Air Temperature  ( °C )" class="XYGraph (strict)"("Y Scale.Display Format:Precision"=u8 2 ("Y Scale.Format & Precision:Precision")) -> ()  [unwired: 2 in, 2 out]
            n2926 = property on="Air Temperature  ( °C )" class="XYGraph (strict)"("X Scale.Range:Minimum"=0.0 ("Y Scale.Range:Minimum"), "X Scale.Range:Maximum"=75.0 ("Y Scale.Range:Maximum"), "Y Scale.Range:Minimum"=20.0 ("X Scale.Range:Minimum"), "Y Scale.Range:Maximum"=26.0 ("X Scale.Range:Maximum")) -> ()  [unwired: 2 in, 2 out]
          }
        }
        n2927 = case shown="True" "RSTV1 4" {
          frame False {
          }
          frame True {
            n2928 = property on="Stroke ( mm )" class="XYGraph (strict)"("Y Scale.Display Format:Precision"=u8 2 ("Y Scale.Format & Precision:Precision")) -> ()  [unwired: 2 in, 2 out]
            n2929 = property on="Stroke ( mm )" class="XYGraph (strict)"("X Scale.Range:Minimum"=0.0 ("Y Scale.Range:Maximum"), "X Scale.Range:Maximum"=75.0 ("X Scale.Range:Minimum"), "Y Scale.Range:Minimum"=0.98, "Y Scale.Range:Maximum"=1.02) -> ()  [unwired: 2 in, 2 out]
          }
        }
        n2930 = case shown="True" "rstv2" {
          frame False {
          }
          frame True {
            n2931 = property on="Coefficient Of Friction" class="XYGraph (strict)"("Y Scale.Display Format:Precision"=u8 3 ("Y Scale.Format & Precision:Precision")) -> ()  [unwired: 2 in, 2 out]
            n2932 = property on="Coefficient Of Friction" class="XYGraph (strict)"("X Scale.Range:Minimum"=0.0 ("Y Scale.Range:Maximum"), "X Scale.Range:Maximum"=75.0, "Y Scale.Range:Minimum"=0.0, "Y Scale.Range:Maximum"=1.0 ("X Scale.Range:Minimum")) -> ()  [unwired: 2 in, 2 out]
          }
        }
        n2933 = case shown="True" "RST CP 3" {
          frame False {
          }
          frame True {
            n2934 = property on="Air Temp ( °C ) vs Humidity ( % RH )" class="XYGraph (strict)"("X Scale.Range:Minimum"=18.0, "X Scale.Range:Maximum"=28.0 ("X Scale.Range:Minimum"), "Y Scale.Range:Minimum"=30.0 ("X Scale.Range:Minimum"), "Y Scale.Range:Maximum"=70.0 ("X Scale.Range:Minimum")) -> ()  [unwired: 2 in, 2 out]
          }
        }
        n2935 = case shown="True" "OPEN 1" {
          frame False {
          }
          frame True {
            (unwired) 0  # existing file
            w3662 = "Choose a datalog file to open"  # prompt
            n2936 = local write "OPEN 1"(FALSE ("OPEN 1")) -> ()
            n2937 = String To Path(string="C:\\LAB-IQ\\Data\\") -> (path=w3647:path)
            n2938 = File Dialog(6:"*.dgf" ("pattern"), 7:w3662, 11:w3647) -> (0:w3645:errorcluster, 3:w3653:path)  [unwired: 4 in, 2 out]
            n2939 = Unbundle(w3645) -> ()  [unwired: 3 out]
            n2940 = Strip Path(path=w3653) -> (name=w3652:string)  [unwired: 1 out]
            n2941 = Path To String(path=w3653) -> (string=w3648:string)
            "string1" <- w3648
            n2942 = Match Pattern(string=w3652, regular expression=".dgf") -> (before substring=→"String Control":string)  [unwired: 1 in, 3 out]
            n2943 = Match Pattern(string=w3648, regular expression=".dgf" ("substring (\"\")")) -> (before substring=w3658:string)  [unwired: 1 in, 3 out]
            n2944 = Concatenate Strings(w3658, ".duf" ("Substring")) -> (w3654:string)
            n2945 = String To Path(string=w3654) -> (path=w3659:path)
            n2946 = call <vilib>:"Read Characters From File.vi"("file path (dialog if empty)"=w3659, "start of read offset (chars.:0)"=60 ("start of read offset (chars.: 0)")) -> ("character string"=→"String Control 2":string)  [unwired: 4 in, 3 out]
          }
        }
        n2947 = case shown="True" "OPEN 2" {
          frame False {
          }
          frame True {
            (unwired) 0  # existing file
            w3680 = "Choose a datalog file to open"  # prompt
            n2948 = local write "OPEN 2"(FALSE ("OPEN 1")) -> ()
            n2949 = String To Path(string="C:\\LAB-IQ\\Data\\") -> (path=w3665:path)
            n2950 = File Dialog(6:"*.dgf" ("pattern"), 7:w3680, 11:w3665) -> (0:w3663:errorcluster, 3:w3671:path)  [unwired: 4 in, 2 out]
            n2951 = Unbundle(w3663) -> ()  [unwired: 3 out]
            n2952 = Strip Path(path=w3671) -> (name=w3669:string)  [unwired: 1 out]
            n2953 = Path To String(path=w3671) -> (string=w3666:string)
            "string1 2" <- w3666
            n2954 = Match Pattern(string=w3669, regular expression=".dgf") -> (before substring=→"String Control 3":string)  [unwired: 1 in, 3 out]
            n2955 = Match Pattern(string=w3666, regular expression=".dgf" ("substring (\"\")")) -> (before substring=w3677:string)  [unwired: 1 in, 3 out]
            n2956 = Concatenate Strings(w3677, ".duf" ("Substring")) -> (w3674:string)
            n2957 = String To Path(string=w3674) -> (path=w3672:path)
            n2958 = call <vilib>:"Read Characters From File.vi"("file path (dialog if empty)"=w3672, "start of read offset (chars.:0)"=60 ("start of read offset (chars.: 0)")) -> ("character string"=→"String Control 4":string)  [unwired: 4 in, 3 out]
          }
        }
        n2959 = case shown="True" "OPEN 3" {
          frame False {
          }
          frame True {
            (unwired) 0  # existing file
            w3698 = "Choose a datalog file to open"  # prompt
            n2960 = local write "OPEN 3"(FALSE ("OPEN 1")) -> ()
            n2961 = String To Path(string="C:\\LAB-IQ\\Data\\") -> (path=w3683:path)
            n2962 = File Dialog(6:"*.dgf" ("pattern"), 7:w3698, 11:w3683) -> (0:w3681:errorcluster, 3:w3689:path)  [unwired: 4 in, 2 out]
            n2963 = Unbundle(w3681) -> ()  [unwired: 3 out]
            n2964 = Strip Path(path=w3689) -> (name=w3687:string)  [unwired: 1 out]
            n2965 = Path To String(path=w3689) -> (string=w3684:string)
            "string1 3" <- w3684
            n2966 = Match Pattern(string=w3687, regular expression=".dgf") -> (before substring=→"String Control 5":string)  [unwired: 1 in, 3 out]
            n2967 = Match Pattern(string=w3684, regular expression=".dgf" ("substring (\"\")")) -> (before substring=w3694:string)  [unwired: 1 in, 3 out]
            n2968 = Concatenate Strings(w3694, ".duf" ("Substring")) -> (w3691:string)
            n2969 = String To Path(string=w3691) -> (path=w3695:path)
            n2970 = call <vilib>:"Read Characters From File.vi"("file path (dialog if empty)"=w3695, "start of read offset (chars.:0)"=60 ("start of read offset (chars.: 0)")) -> ("character string"=→"String Control 6":string)  [unwired: 4 in, 3 out]
          }
        }
        n2971 = case shown="True" "OPEN 4" {
          frame False {
          }
          frame True {
            (unwired) 0  # existing file
            w3716 = "Choose a datalog file to open"  # prompt
            n2972 = local write "OPEN 4"(FALSE ("OPEN 1")) -> ()
            n2973 = String To Path(string="C:\\LAB-IQ\\Data\\") -> (path=w3701:path)
            n2974 = File Dialog(6:"*.dgf" ("pattern"), 7:w3716, 11:w3701) -> (0:w3699:errorcluster, 3:w3707:path)  [unwired: 4 in, 2 out]
            n2975 = Unbundle(w3699) -> ()  [unwired: 3 out]
            n2976 = Strip Path(path=w3707) -> (name=w3705:string)  [unwired: 1 out]
            n2977 = Path To String(path=w3707) -> (string=w3702:string)
            "string1 4" <- w3702
            n2978 = Match Pattern(string=w3705, regular expression=".dgf") -> (before substring=→"String Control 7":string)  [unwired: 1 in, 3 out]
            n2979 = Match Pattern(string=w3702, regular expression=".dgf" ("substring (\"\")")) -> (before substring=w3712:string)  [unwired: 1 in, 3 out]
            n2980 = Concatenate Strings(w3712, ".duf" ("Substring")) -> (w3709:string)
            n2981 = String To Path(string=w3709) -> (path=w3713:path)
            n2982 = call <vilib>:"Read Characters From File.vi"("file path (dialog if empty)"=w3713, "start of read offset (chars.:0)"=60 ("start of read offset (chars.: 0)")) -> ("character string"=→"String Control 8":string)  [unwired: 4 in, 3 out]
          }
        }
      }
      frame "About" {
        # "Elapsed time\ncof\nstroke\nmean pos\nTemp\nHumidity"
        n2983 = disable-structure shown="Disabled" {
          frame Disabled {
            n2984 = case shown="True" "Export" {
              frame False {
              }
              frame True {
                w3738 = "                                      " ("string")
                w3740 = "\r"
                (unwired) i16 6 ("width (-)")
                w3817 = "\r"
                w3749 = "\r"
                n2985 = local write "Export"(FALSE ("Export")) -> ()
                n2986 = local read "String 29"() -> (w3786:string)
                n2987 = local read "String 34"() -> (w3774:string)
                n2988 = local read "String 35"() -> (w3769:string)
                n2989 = local read "String 37"() -> (w3765:string)
                n2990 = local read "String 36"() -> (w3762:string)
                n2991 = local read "String 38"() -> (w3759:string)
                n2992 = local read "String 39"() -> (w3756:string)
                n2993 = Match Pattern(string=w3786, regular expression=".dwm") -> (before substring=w3782:string)  [unwired: 1 in, 3 out]
                "before substring" <- w3782
                n2994 = local read "S 38"() -> (w3777:string)
                n2995 = local read "S 39"() -> (w3770:string)
                n2996 = local read "Temperature before test 2"() -> (w3806:dbl)
                n2997 = local read "Temperature after test 2"() -> (w3811:dbl)
                n2998 = local read "Humidity before test 2"() -> (w3792:dbl)
                n2999 = local read "Humidity after test 2"() -> (w3807:dbl)
                n3000 = local read "MWSD 2"() -> (w3803:dbl)
                n3001 = local read "WS1.4 2"() -> (w3819:dbl)
                n3002 = local read "HCF 2"() -> (w3815:dbl)
                n3003 = local read "AVP 2"() -> (w3804:dbl)
                n3004 = Concatenate Strings("1," ("string"), w3777) -> (w3776:string)
                n3005 = Concatenate Strings("2," ("string"), w3774) -> (w3773:string)
                n3006 = Concatenate Strings("3," ("string"), w3770) -> (w3772:string)
                n3007 = Concatenate Strings("4," ("string"), w3769) -> (w3768:string)
                n3008 = Concatenate Strings("5," ("string"), w3765) -> (w3766:string)
                n3009 = Concatenate Strings("6," ("string"), w3762) -> (w3763:string)
                n3010 = Concatenate Strings("7," ("string"), w3759) -> (w3760:string)
                n3011 = Concatenate Strings("8," ("string"), w3756) -> (w3757:string)
                n3012 = local read "Sample ID"() -> (w3824:string)
                n3013 = case shown="\"xlx\"" "Select File Type" {
                  tunnel: w3782 -> [w3827 w3829 w3831]
                  tunnel: [w3825 w3830 w3832] -> w3781
                  frame "xlx" {
                    n3014 = Concatenate Strings(w3827, ".xls" ("string")) -> (w3825:string)
                  }
                  frame "csv" {
                    n3015 = Concatenate Strings(w3829, ".csv" ("string")) -> (w3830:string)
                  }
                  frame "txt" {
                    n3016 = Concatenate Strings(w3831, ".txt" ("string")) -> (w3832:string)
                  }
                }
                n3017 = local read "Test Date"() -> (w3823:string)
                n3018 = local read "String 45"() -> (w3737:string)
                n3019 = local read "String 31"() -> (w3822:string)
                n3020 = local read "String 32"() -> (w3821:string)
                n3021 = local read "TITTLE"() -> (w3745:string)
                n3022 = Number To Fractional String(number=w3792, width (-)=i16 6, precision (6)=i16 2) -> (F-format string=w3791:string)  [unwired: 1 in]
                n3023 = Number To Fractional String(number=w3806, width (-)=i16 6, precision (6)=i16 2) -> (F-format string=w3812:string)  [unwired: 1 in]
                n3024 = Number To Fractional String(number=w3807, width (-)=i16 6, precision (6)=i16 2) -> (F-format string=w3805:string)  [unwired: 1 in]
                n3025 = Number To Fractional String(number=w3811, width (-)=i16 6, precision (6)=i16 2) -> (F-format string=w3810:string)  [unwired: 1 in]
                n3026 = Number To Fractional String(number=w3803, width (-)=i16 6, precision (6)=i16 2) -> (F-format string=w3801:string)  [unwired: 1 in]
                n3027 = Number To Fractional String(number=w3804, width (-)=i16 6, precision (6)=i16 2) -> (F-format string=w3802:string)  [unwired: 1 in]
                n3028 = Number To Fractional String(number=w3815, width (-)=i16 6, precision (6)=i16 2) -> (F-format string=w3816:string)  [unwired: 1 in]
                n3029 = Number To Fractional String(number=w3819, precision (6)=i16 2) -> (F-format string=w3820:string)  [unwired: 2 in]
                n3030 = local read "s.NO"() -> (w3739:string)
                n3031 = Concatenate Strings("=" ("string"), w3745) -> (w3744:string)
                n3032 = Concatenate Strings("S.No," ("string"), "                                       Parameters" ("string")) -> (w3750:string)
                n3033 = Concatenate Strings(w3817, w3776, w3791, w3817, w3773, w3812, w3817, w3772, w3805, w3817, w3768, w3810, w3817, w3766, w3801, w3817, w3763, w3802, w3817, w3760, w3816, w3817, w3757, w3820) -> (w3779:string)
                n3034 = Concatenate Strings(w3749, "," ("string"), w3737, w3739, w3738, w3821, w3824, w3738, w3822, w3823, w3749) -> (w3747:string)
                n3035 = local read "Tested by"() -> (w3753:string)
                n3036 = local read "String 33"() -> (w3754:string)
                n3037 = Concatenate Strings("," ("string"), "                                                                             " ("string")) -> (w3742:string)
                n3038 = Concatenate Strings(w3744, w3740, w3747, w3740, w3750, w3779, w3740, w3742, w3754, w3753) -> (→"export":string)
                n3039 = String To Path(string=w3781) -> (path=w3788:path)
                n3040 = local read "export"() -> (w3783:string)
